vi "Table_Put_Resultes_and_Decided_Pass_Fail.vi"(0 "Result 2":dbl=nan, 1 "Result 1 Array":dbl[](array[numeric]), 2 "Result 1":dbl=nan, 3 "Test Paragraph":string="4.4.1", 5 "Result 2 Array":dbl[](array[numeric]), 7 "Result 3":dbl=nan, 9 "Result 3 Array":dbl[](array[numeric]), 11 "Error in":errorcluster, 12 "Array of data-array\ncluster (instead the 3\n \"Results Array\")":cluster{"Result Array":dbl[]}[](array[cluster]), 13 "Array of Data\n(instead the 3\n \"Results\")":dbl[](array[numeric]), 14 "Table Ref.":refnum<vi>) -> (4 "Pass/Fail":bool, 8 "Table Ref. Out":refnum<vi>, 10 "Table Out":string[][](table)=[["Led -Test & On/Rst.Msg.", "", "", "", "", "", "", "", "", " ", "", "", "", "", " "], ["Led Test", "", "#1", "-", "-", "", "", "", "", " ", "", "", "", "", ""], ["Com.RS232 Rst.Msg", "", "#2", "-", "-", "", "", "", "", " ", "", "", "", "", ""], ["Com.RS232 Ans.Msg", "", "#3", "-", "-", "", "", "", "", "", "", "", "", "", ""], ["", "", "", "", "", "", "", "", "", "", "", "", "", "", ""], ["Servo Voltage & Current", "", "", "", "", "", "", "", "FAIL", "", "", "", "", "", ""], ["Servo Voltage", "", "28.0", "+/-1", "V", "", "NaN", "", "FAIL", "", "6.0", "0.0", "100", "Average", ""], ["Servo Current", "", "0.15", "Max", "A", "", "NaN", "", "FAIL", "", "1.0", "0.0", "100", "Average", ""], ["", "", "", "", "", "", "", "", "", "", "", "", "", "", ""], ["Voltages Accurance", "", "", "", "", "", "", "", "FAIL", "", "", "", "", "", ""], ["Servo VCC 5V    ", "", "5.0", "+/-0.1", "V", "", "NaN", "", "FAIL", "", "1.0", "0.0", "100", "Average", ""], ["Servo VEE -6.8V", "", "-6.8", "+/-0.15", "V", "", "NaN", "", "FAIL", "", "1.0", "0.0", "100", "Average", ""], ["Ref_1_4.096V ?", "", "4.096", "+/-0.1", "V", "", "NaN", "", "FAIL", "", "1.0", "0.0", "100", "Average", ""], ["", "", "", "", "", "", "", "", "", "", "", "", "", "", ""], ["Power-Supply Changing", "", "", "", "", "", "", "", "", "", "", "", "", "", ""], ["Min. Power-Supply Volt. 18v ", "", "Led Flashes", "-", "-", "", "", "", "", "", "", "", "", "", ""], ["Max. Power-Supply Volt. 32v ", "", "Led Flashes", "-", "-", "", "", "", "", "", "", "", "", "", ""], ["Under Volt.Prot.28->5->18v", "", "Led Flashes", "-", "-", "", "", "", "", "", "", "", "", "", ""], ["", "", "", "", "", "", "", "", "", "", "", "", "", "", ""], ["Pos.Cmd.Accur.@Mode1", "", "Mxxxx=", "", "", "", "", "", "", "", "", "", "", "", ""], ["Pos.Cmnd.=0.5V F.B.", "", "59h", "+/-5", "", "", "", "", "", "", "1.0", "0.0", "1", "Average", ""], ["Pos.Cmnd.=2.0V F.B.", "", "195h", "+/-5", "", "", "", "", "", "", "1.0", "0.0", "1", "Average", ""], ["Pos.Cmnd.=4.5V F.B.", "", "3A5h", "+/-5", "", "", "", "", "", "", "1.0", "0.0", "1", "Average", ""], ["", "", "", "", "", "", "", "", "", "", "", "", "", "", ""], ["Pos.Cmd.Accur.@Mode2", "", "Mxxxx=", "", "", "", "", "", "FAIL", "", "", "", "", "", ""], ["Pos.Cmnd.=0.5V F.B", "", "59h", "+/-5", "", "", "57h", "", "PASS", "", "1.0", "0.0", "1", "Average", ""], ["Pos.Cmnd.=2.0V F.B.", "", "195h", "+/-5", "", "", "1CEh", "", "FAIL", "", "1.0", "0.0", "1", "Average", ""], ["Pos.Cmnd.=4.5V F.B.", "", "3A5h", "+/-5", "", "", "2BAh", "", "FAIL", "", "1.0", "0.0", "1", "Average", ""], ["", "", "", "", "", "", "", "", "", "", "", "", "", "", ""], ["Pot.Accur.@Mode1 ", "", "Rxxxx=", "", "", "", "", "", "FAIL", "", "", "", "", "", ""], ["Pot.simulate=0.5v Pot.Code.:", "", "173h", "+/-5", "", "", "7Bh", "", "FAIL", "", "1.0", "0.0", "1", "Average", ""], ["Pot.simulate=2.0v Pot.Code.:", "", "1F3h", "+/-5", "", "", "1F1h", "", "PASS", "", "1.0", "0.0", "1", "Average", ""], ["Pot.simulate=3.5v Pot.Code.:", "", "372h", "+/-5", "", "", "368h", "", "FAIL", "", "1.0", "0.0", "1", "Average", ""], ["", "", "", "", "", "", "", "", "", "", "", "", "", "", ""], ["Pot.Accur.@Mode2 ", "", "Rxxxx=", "", "", "", "", "", "FAIL", "", "", "", "", "", ""], ["Pot.simulate=0.5v Pot.Code.:", "", "C4h", "+/-5", "", "", "7Bh", "", "FAIL", "", "1.0", "0.0", "1", "Average", ""], ["Pot.simulate=2.0v Pot.Code.:", "", "1E3h", "+/-5", "", "", "1F1h", "", "FAIL", "", "1.0", "0.0", "1", "Average", ""], ["Pot.simulate=3.5v Pot.Code.:", "", "541h", "+/-5", "", "", "368h", "", "FAIL", "", "1.0", "0.0", "1", "Average", ""], ["", "", "", "", "", "", "", "", "", "", "", "", "", "", ""], ["Status Accur.@Mode1", "", "", "", "", "", "", "", "", "", "", "", "", "", ""], ["Pot. / Pos.Cmnd. 1.5v", "", "-1.8084", "+/-0.1", "V", "", "", "", "", "", "1.0", "0.0", "100", "Average", ""], ["Pot. / Pos.Cmnd. 2.0v", "", "-0.1584", "+/-0.1", "V", "", "", "", "", "", "1.0", "0.0", "100", "Average", ""], ["Pot. / Pos.Cmnd. 3.5v", "", "4.7916", "+/-0.1", "V", "", "", "", "", "", "1.0", "0.0", "100", "Average", ""]], 15 "Error out":errorcluster)   [LabVIEW 2017]
panel:
  out "Table In":string[][](table)=[["Led -Test & On/Rst.Msg.", "", "", "", "", "", "", "", "", " ", "", "", "", "", " "], ["Led Test", "", "#1", "-", "-", "", "", "", "", " ", "", "", "", "", ""], ["Com.RS232 Rst.Msg", "", "#2", "-", "-", "", "", "", "", " ", "", "", "", "", ""], ["Com.RS232 Ans.Msg", "", "#3", "-", "-", "", "", "", "", "", "", "", "", "", ""], ["", "", "", "", "", "", "", "", "", "", "", "", "", "", ""], ["Servo Voltage & Current", "", "", "", "", "", "", "", "FAIL", "", "", "", "", "", ""], ["Servo Voltage", "", "28.0", "+/-1", "V", "", "NaN", "", "FAIL", "", "6.0", "0.0", "100", "Average", ""], ["Servo Current", "", "0.15", "Max", "A", "", "NaN", "", "FAIL", "", "1.0", "0.0", "100", "Average", ""], ["", "", "", "", "", "", "", "", "", "", "", "", "", "", ""], ["Voltages Accurance", "", "", "", "", "", "", "", "FAIL", "", "", "", "", "", ""], ["Servo VCC 5V    ", "", "5.0", "+/-0.1", "V", "", "NaN", "", "FAIL", "", "1.0", "0.0", "100", "Average", ""], ["Servo VEE -6.8V", "", "-6.8", "+/-0.15", "V", "", "NaN", "", "FAIL", "", "1.0", "0.0", "100", "Average", ""], ["Ref_1_4.096V ?", "", "4.096", "+/-0.1", "V", "", "NaN", "", "FAIL", "", "1.0", "0.0", "100", "Average", ""], ["", "", "", "", "", "", "", "", "", "", "", "", "", "", ""], ["Power-Supply Changing", "", "", "", "", "", "", "", "", "", "", "", "", "", ""], ["Min. Power-Supply Volt. 18v ", "", "Led Flashes", "-", "-", "", "", "", "", "", "", "", "", "", ""], ["Max. Power-Supply Volt. 32v ", "", "Led Flashes", "-", "-", "", "", "", "", "", "", "", "", "", ""], ["Under Volt.Prot.28->5->18v", "", "Led Flashes", "-", "-", "", "", "", "", "", "", "", "", "", ""], ["", "", "", "", "", "", "", "", "", "", "", "", "", "", ""], ["Pos.Cmd.Accur.@Mode1", "", "Mxxxx=", "", "", "", "", "", "", "", "", "", "", "", ""], ["Pos.Cmnd.=0.5V F.B.", "", "59h", "+/-5", "", "", "", "", "", "", "1.0", "0.0", "1", "Average", ""], ["Pos.Cmnd.=2.0V F.B.", "", "195h", "+/-5", "", "", "", "", "", "", "1.0", "0.0", "1", "Average", ""], ["Pos.Cmnd.=4.5V F.B.", "", "3A5h", "+/-5", "", "", "", "", "", "", "1.0", "0.0", "1", "Average", ""], ["", "", "", "", "", "", "", "", "", "", "", "", "", "", ""], ["Pos.Cmd.Accur.@Mode2", "", "Mxxxx=", "", "", "", "", "", "FAIL", "", "", "", "", "", ""], ["Pos.Cmnd.=0.5V F.B", "", "59h", "+/-5", "", "", "57h", "", "PASS", "", "1.0", "0.0", "1", "Average", ""], ["Pos.Cmnd.=2.0V F.B.", "", "195h", "+/-5", "", "", "1CEh", "", "FAIL", "", "1.0", "0.0", "1", "Average", ""], ["Pos.Cmnd.=4.5V F.B.", "", "3A5h", "+/-5", "", "", "2BAh", "", "FAIL", "", "1.0", "0.0", "1", "Average", ""], ["", "", "", "", "", "", "", "", "", "", "", "", "", "", ""], ["Pot.Accur.@Mode1 ", "", "Rxxxx=", "", "", "", "", "", "FAIL", "", "", "", "", "", ""], ["Pot.simulate=0.5v Pot.Code.:", "", "173h", "+/-5", "", "", "7Bh", "", "FAIL", "", "1.0", "0.0", "1", "Average", ""], ["Pot.simulate=2.0v Pot.Code.:", "", "1F3h", "+/-5", "", "", "1F1h", "", "PASS", "", "1.0", "0.0", "1", "Average", ""], ["Pot.simulate=3.5v Pot.Code.:", "", "372h", "+/-5", "", "", "368h", "", "FAIL", "", "1.0", "0.0", "1", "Average", ""], ["", "", "", "", "", "", "", "", "", "", "", "", "", "", ""], ["Pot.Accur.@Mode2 ", "", "Rxxxx=", "", "", "", "", "", "FAIL", "", "", "", "", "", ""], ["Pot.simulate=0.5v Pot.Code.:", "", "C4h", "+/-5", "", "", "7Bh", "", "FAIL", "", "1.0", "0.0", "1", "Average", ""], ["Pot.simulate=2.0v Pot.Code.:", "", "1E3h", "+/-5", "", "", "1F1h", "", "FAIL", "", "1.0", "0.0", "1", "Average", ""], ["Pot.simulate=3.5v Pot.Code.:", "", "541h", "+/-5", "", "", "368h", "", "FAIL", "", "1.0", "0.0", "1", "Average", ""], ["", "", "", "", "", "", "", "", "", "", "", "", "", "", ""], ["Status Accur.@Mode1", "", "", "", "", "", "", "", "", "", "", "", "", "", ""], ["Pot. / Pos.Cmnd. 1.5v", "", "-1.8084", "+/-0.1", "V", "", "", "", "", "", "1.0", "0.0", "100", "Average", ""], ["Pot. / Pos.Cmnd. 2.0v", "", "-0.1584", "+/-0.1", "V", "", "", "", "", "", "1.0", "0.0", "100", "Average", ""], ["Pot. / Pos.Cmnd. 3.5v", "", "4.7916", "+/-0.1", "V", "", "", "", "", "", "1.0", "0.0", "100", "Average", ""]]
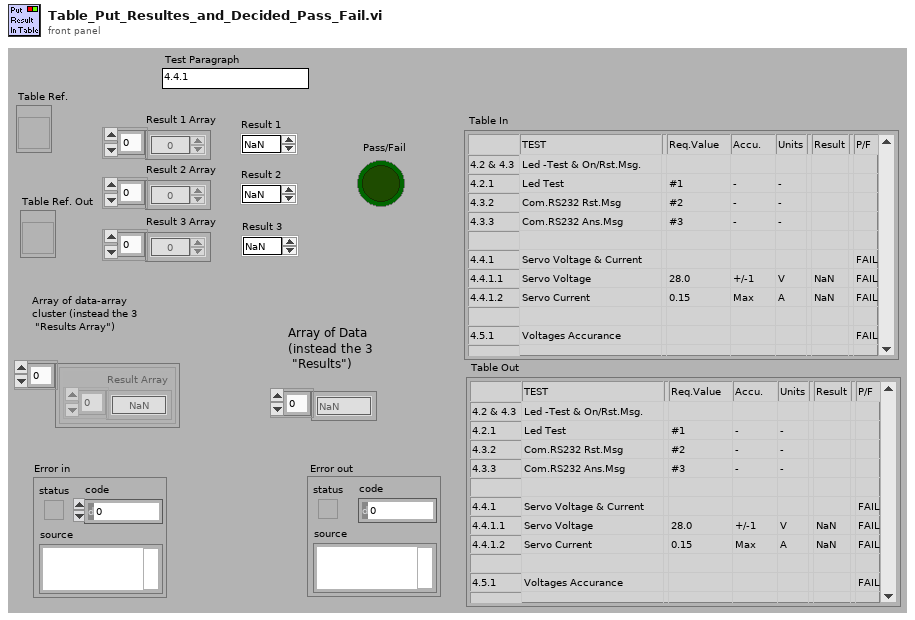
[diagram p1: front panel]
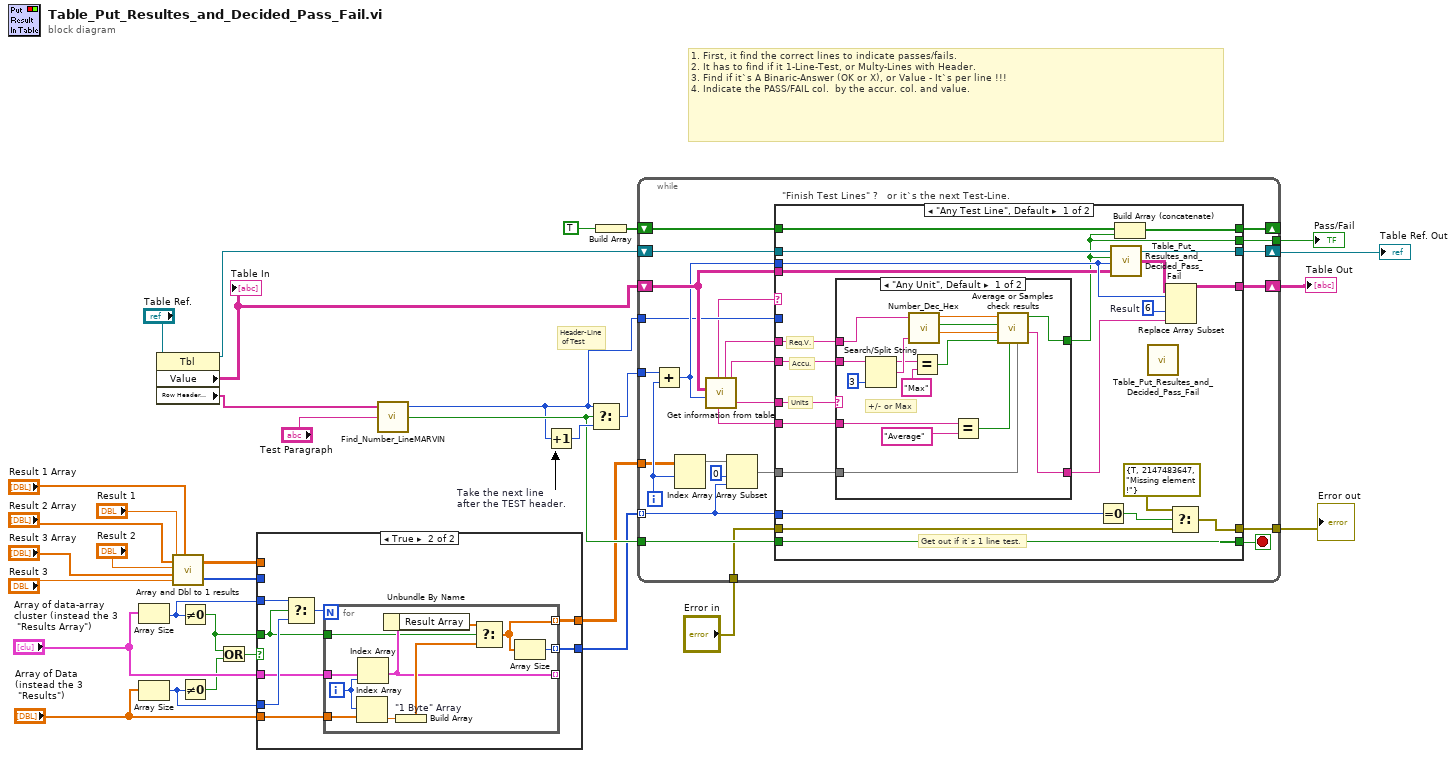
[diagram p0: block diagram]
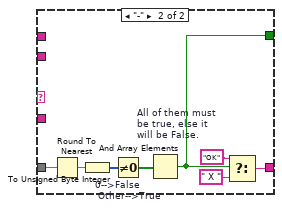
[diagram p3: hidden frame]
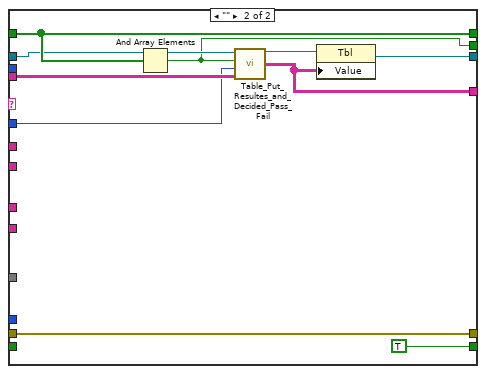
[diagram p4: hidden frame]
diagram:
  # "Header-Line\n of Test"
  # "1. First, it find the correct lines to indicate passes/fails.\n2. It has to find if it 1-Line-Test, or Multy-Lines with Header.\n3. Find if it`s A Binaric-Answer (OK or X), or Value - It`s per line !!!\n4. Indicate the PASS/FAIL col.  by the accur. col. and value."
  n1 = Array Size(array="Array of data-array\ncluster (instead the 3\n \"Results Array\")") -> (size(s)=w7:i32)
  n2 = Array Size(array="Array of Data\n(instead the 3\n \"Results\")") -> (size(s)=w6:i32)
  n3 = property class="Tbl"(reference="Table Ref.") -> (reference out=w28:refnum<vi>, "Value"=w27:string[][], "Row Header Strings[]"=w31:string[])  [unwired: 1 in, 1 out]
  "Table In" <- w27
  n4 = call "Array and Dbl to 1 results.vi"("Result3"="Result 3", "Result 1 Array"="Result 1 Array", "Result 3 Array"="Result 3 Array", "Result2"="Result 2", "Result 2 Array"="Result 2 Array", "Result1"="Result 1") -> ("Length"=w12:i32[], "Array Set"=w14:dbl[][])
  n5 = Not Equal To 0?(x=w7) -> (x != 0?=w4:bool)
  n6 = Not Equal To 0?(x=w6) -> (x != 0?=w5:bool)
  n7 = Or(x=w4, y=w5) -> (x .or. y?=w8:bool)
  n8 = case shown="True" w8 {
    tunnel: w14 -> [w35 _]
    tunnel: [w35 w43] -> w13
    tunnel: w12 -> [w34 _]
    tunnel: [w34 w42] -> w11
    tunnel: "Array of Data\n(instead the 3\n \"Results\")" -> [_ w37]
    tunnel: "Array of data-array\ncluster (instead the 3\n \"Results Array\")" -> [_ w38]
    tunnel: w7 -> [_ w41]
    tunnel: w6 -> [_ w40]
    tunnel: w4 -> [_ w36]
    frame False {
    }
    frame True {
      n9 = Select(t=w41, s=w36, f=w40) -> (s? t:f=w39:i32)
      n10 = for {
        N: w39 -> [_]
        tunnel: w38 -> [w49]
        tunnel: [w48] -> _ mode=indexing
        tunnel: [w52] -> w43 mode=indexing
        tunnel: [w53] -> w42 mode=indexing
        tunnel: w37 -> [w47]
        tunnel: w36 -> [w44]
        i -> [w46]
        n11 = Index Array(array=w47, index=w46) -> (element=w45:dbl)
        n12 = Index Array(array=w49, index=w46) -> (element=w48:cluster{"Result Array":dbl[]})
        n13 = Unbundle By Name(w48) -> ("Result Array"=w50:dbl[])
        n14 = Build Array "\"1 Byte\" Array"(w45) -> (w51:dbl[])
        n15 = Select(t=w50, s=w44, f=w51) -> (s? t:f=w52:dbl[])
        n16 = Array Size(array=w52) -> (size(s)=w53:i32)
      }
    }
  }
  n17 = call "Find_Number_LineMARVIN.vi"("Test Paragraph"="Test Paragraph", "Row Headers[]"=w31) -> ("1 line Test ?"=w23:bool, "Line number"=w22:i32)  [unwired: 1 in, 1 out]
  n18 = Increment "Take the next line \nafter the TEST header."(x=w22) -> (x+1=w30:i32)
  n19 = Select(t=w22, s=w23, f=w30) -> (s? t:f=w29:i32)
  n20 = Build Array(TRUE) -> (w24:bool[])
  n21 = while {
    tunnel: w29 -> [w77]
    shift-right: [w73] -> w26
    shift-left: w27 -> [w74]
    shift-right: [w71] -> w1
    shift-left: w28 -> [w70]
    shift-right: [w68] -> _
    shift-left: w24 -> [w69]
    tunnel: w23 -> [w67]
    tunnel: w22 -> [w66]
    tunnel: [w65] -> w21
    tunnel: w13 -> [w62]
    tunnel: w11 -> [w54] mode=indexing
    tunnel: [w56] -> w2
    tunnel: "Error in" -> [w55]
    i -> [w64]
    stop <- w78 stop-if-true
    n22 = Add(x=w77, y=w64) -> (x+y=w72:i32)
    n23 = Index Array(array=w62, index (row)=w64) -> (element=w61:dbl[])  [unwired: 1 in]
    n24 = call "Get information from table.vi"("Numeric"=w72, "Table"=w74) -> ("Average/Samples"=w57:string, "Units"=w76:string, "Test Name"=w59:string, "Request Value"=w58:string, "Accurrance"=w75:string)  [unwired: 2 in, 3 out]
    n25 = Array Subset(array=w61, index=0, length=w54) -> (w63:dbl[])
    n26 = case "\"Finish Test Lines\" ?   or it`s the next Test-Line." shown="\"Any Test Line\", Default" w59 {
      tunnel: w76 -> [w100 _]
      tunnel: [w93 TRUE] -> w78
      tunnel: w75 -> [w99 _]
      tunnel: w58 -> [w98 _]
      tunnel: w74 -> [w89 w130]
      tunnel: [w88 w125] -> w73
      tunnel: w72 -> [w90 _]
      tunnel: w70 -> [w91 w128]
      tunnel: [w92 w133] -> w71
      tunnel: w69 -> [w95 w132]
      tunnel: [w94 w132] -> w68
      tunnel: w67 -> [w93 _]
      tunnel: w66 -> [_ w129]
      tunnel: [w87 w127] -> w65
      tunnel: w63 -> [w86 _]
      tunnel: w57 -> [w85 _]
      tunnel: [w81 w126] -> w56
      tunnel: w55 -> [w82 w126]
      tunnel: w54 -> [w84 _]
      frame "Any Test Line", Default {
        w97 = 6  # Result
        # "Get out if it`s 1 line test."
        # "Accu."
        # "Req.V."
        # "Units"
        n27 = case shown="\"Any Unit\", Default" w100 {
          tunnel: [w104 w120] -> w96
          tunnel: [w105 w117] -> w87
          tunnel: w99 -> [w115 _]
          tunnel: w98 -> [w108 _]
          tunnel: w86 -> [w106 w119]
          tunnel: w85 -> [w103 _]
          frame "Any Unit", Default {
            # "+/- or Max"
            n28 = Search/Split String(string=w115, offset (0)=3) -> (substring before match=w111:string, match + rest of string=w112:string)  [unwired: 1 in, 1 out]
            n29 = call "Number_Dec_Hex.vi"("Dec(Any)/Hex(unsigned only) Number"=w108, "Dec(Any)/Hex(unsigned only) Number 2"=w112) -> ("Numeric"=w116:dbl, "Dec (True) or\nHex (False)"=w107:bool, "Numeric 2"=w109:dbl)  [unwired: 1 in, 3 out]
            n30 = Equal?(x=w111, y="Max") -> (x = y?=w114:bool)
            n31 = Equal?(x=w103, y="Average") -> (x = y?=w101:bool)
            n32 = call "Average or Samples check results.vi"("Array"=w106, "Average(True)\nor Samples(False)"=w101, "In Range (True)\nor Max (False)"=w114, "Accurrance.\n(unused for Max check)"=w109, "Dec (True) or\nHex (False)"=w107, "Value (or Max value)"=w116) -> ("String"=w104:string, "Results OK ?"=w105:bool)  [unwired: 4 in]
          }
          frame "-" {
            n33 = Round To Nearest(number=w119) -> (nearest integer value=w124:dbl[])
            n34 = To Unsigned Byte Integer(number=w124) -> (unsigned 8bit integer=w123:u8[])
            n35 = Not Equal To 0? "0-->False\n Other-->True"(x=w123) -> (x != 0?=w118:bool[])
            n36 = And Array Elements "All of them must\nbe true, else it\nwill be False."(Boolean array=w118) -> (logical AND=w117:bool)
            n37 = Select(t="OK", s=w117, f=" X ") -> (s? t:f=w120:string)
          }
        }
        n38 = Equal To 0?(x=w84) -> (x = 0?=w83:bool)
        n39 = call "Table_Put_Resultes_and_Decided_Pass_Fail.vi"("Table In"=w89, "Line in table"=w90, "Pass(T) / Fail(F)"=w87, "Table Ref. in"=w91) -> ("Table Out"=w79:string[][], "Table Ref. out"=w92:refnum<vi>)  [unwired: 1 in]
        n40 = Build Array (concatenate)(w95, w87) -> (w94:bool[])
        n41 = call "Table_Put_Resultes_and_Decided_Pass_Fail.vi"() -> ()  [unwired: 12 in, 4 out]
        n42 = Replace Array Subset(array=w79, new element=w96, index (row)=w90, index (col)=w97) -> (w88:string[][])
        n43 = Select(t=errorcluster {"status"=TRUE, "code"=2147483647, "source"="Missing element !"}, s=w83, f=w82) -> (s? t:f=w81:errorcluster)
      }
      frame "" {
        n44 = And Array Elements(Boolean array=w132) -> (logical AND=w127:bool)
        n45 = call "Table_Put_Resultes_and_Decided_Pass_Fail.vi"("Table In"=w130, "Line in table"=w129, "Pass(T) / Fail(F)"=w127, "Table Ref. in"=w128) -> ("Table Out"=w125:string[][], "Table Ref. out"=w131:refnum<vi>)  [unwired: 1 in]
        n46 = property class="Tbl"(reference=w131, "Value"=w125) -> (reference out=w133:refnum<vi>)  [unwired: 1 in, 1 out]
      }
    }
  }
  "Error out" <- w2
  "Table Out" <- w26
  "Pass/Fail" <- w21
  "Table Ref. Out" <- w1
